vi "Special Replace of SubVI Node.vi"(6 "GObj Label":string, 8 "error in (no error)":errorcluster, 9 "Case Insensitive Match? (F)":bool, 10 "Class Path":path, 11 "vi reference in":refnum<vi>) -> (0 "error out":errorcluster, 2 "Replace":refnum<vi>, 3 "vi reference out":refnum<vi>)   [LabVIEW 2020, in "Message Maker.lvlib"]
uses:
  Message Maker.lvlib
  <vilib>/Utility/traverseref.llb/TRef TravTarget.ctl
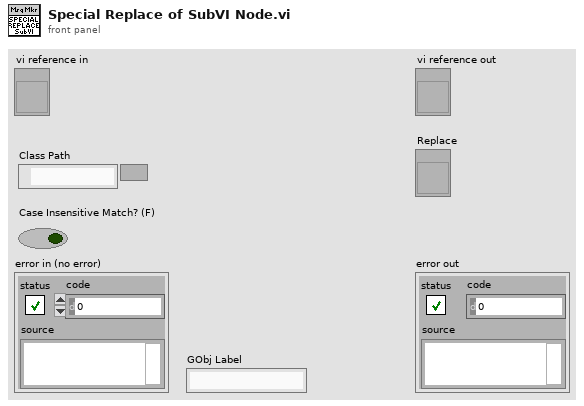
[diagram p1: front panel]
types:
  T1 = typedef "TRef TravTarget.ctl" = enum16{"FP", "BD", "Other"}
  T2 = typedef "LVPositionTypeDef.ctl" = cluster{"Left":i32, "Top":i32}
  T3 = typedef "LVBoundsTypeDef.ctl" = cluster{"Width":u32, "Height":u32}
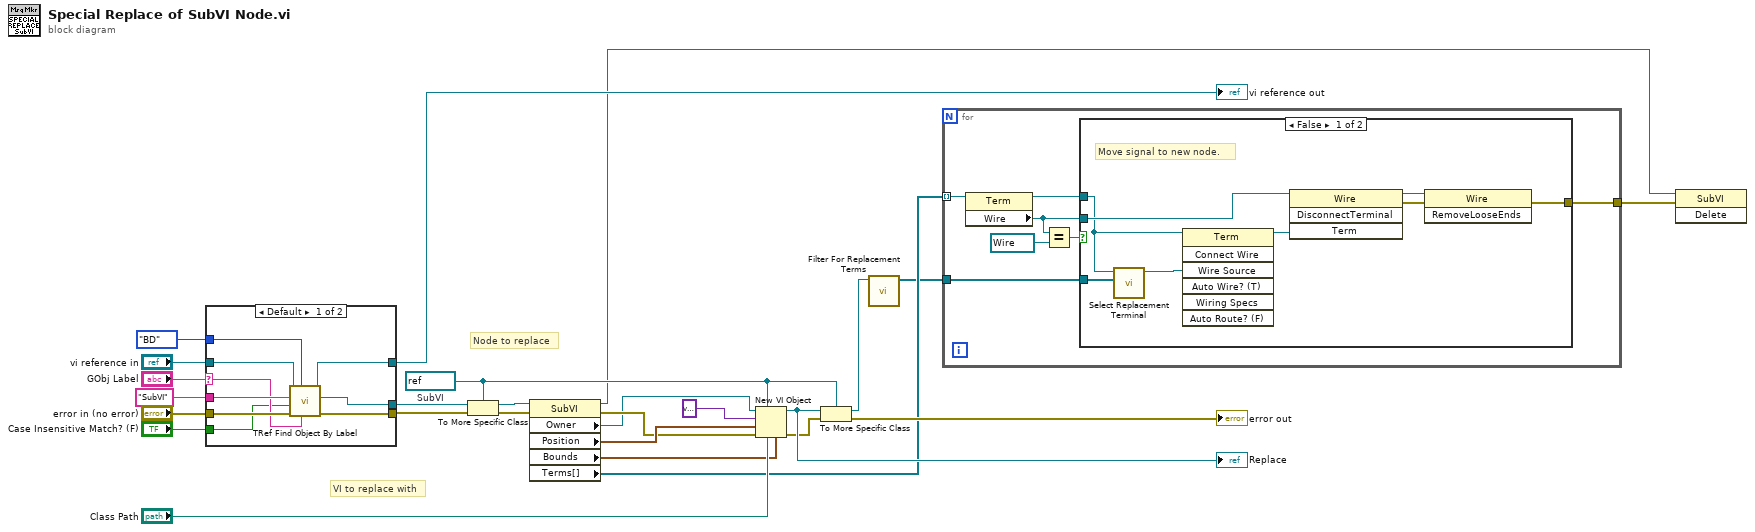
[diagram p0: block diagram]
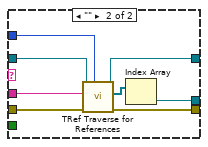
[diagram p2: hidden frame]
diagram:
  w7 = refnum<vi> refnum  # SubVI
  # "VI to replace with"
  # "Node to replace"
  n1 = case shown="Default" "GObj Label" {
    selector: "GObj Label" -> [w29 _]
    tunnel: [w34 w43] -> w17
    tunnel: [w28 w42] -> w19
    tunnel: "SubVI" ("GObj Class Name") -> [w30 w40]
    tunnel: TRef_TravTarget."BD" ("Traverse Target") -> [w33 w39]
    tunnel: [w31 w38] -> w24
    tunnel: "vi reference in" -> [w32 w37]
    tunnel: "error in (no error)" -> [w35 w36]
    tunnel: "Case Insensitive Match? (F)" -> [w27 _]
    frame Default {
      n2 = call <vilib>:"TRef Find Object By Label.vi"("Label"=w29, "Traverse Target"=w33, "error in (no error)"=w35, "Case Insensitive Match? (F)"=w27, "Class Name"=w30, "VI Ref"=w32) -> ("error out"=w34:errorcluster, "Found Obj Ref"=w28:refnum<vi>, "dup VI Ref"=w31:refnum<vi>)  [unwired: 2 in, 1 out]
    }
    frame "" {
      n3 = call <vilib>:"TRef Traverse for References.vi"("Traverse Target"=w39, "error in (no error)"=w36, "Class Name"=w40, "VI Refnum"=w37) -> ("error out"=w43:errorcluster, "References"=w41:refnum<vi>[], "dup VI Refnum"=w38:refnum<vi>)  [unwired: 4 in, 1 out]
      n4 = Index Array(array=w41) -> (element=w42:refnum<vi>)  [unwired: 1 in]
    }
  }
  "vi reference out" <- w24
  n5 = To More Specific Class(target class=w7, reference=w19, error in=w17) -> (specific class reference=w18:refnum<vi>, error out=w16:errorcluster)
  n6 = property class="SubVI"(reference=w18, error in=w16) -> (reference out=w2:refnum<vi>, error out=w15:errorcluster, "Owner"=w13:refnum<vi>, "Position"=w20:T2, "Bounds"=w11:T3, "Terms[]"=w6:refnum<vi>[])
  n7 = New VI Object(vi object class=w7, owner refnum=w13, style=variant, position/next to=w20, 4:w11, 6:"Class Path", 8:w15) -> (object refnum=w10:refnum<vi>, 0:w9:errorcluster)  [unwired: 1 in]
  "Replace" <- w10
  n8 = To More Specific Class(target class=w7, reference=w10, error in=w9) -> (specific class reference=w5:refnum<vi>, error out=→"error out":errorcluster)
  n9 = call "Filter For Replacement Terms.vi"("SubVI in"=w5) -> ("Terms[]"=w4:refnum<vi>[])  [unwired: 10 in]
  n10 = for {
    tunnel: w6 -> [w50] mode=indexing
    tunnel: w4 -> [w46]
    tunnel: [w44] -> w3
    n11 = property class="Term"(reference=w50) -> (reference out=w47:refnum<vi>, "Wire"=w45:refnum<vi>)  [unwired: 1 in, 1 out]
    n12 = Equal?(x=w45, y=refnum<vi> refnum ("Connected Wire")) -> (x = y?=w48:bool)
    n13 = case shown="False" w48 {
      tunnel: w47 -> [w51 _]
      tunnel: w46 -> [w58 _]
      tunnel: w45 -> [w57 _]
      tunnel: [w52 _] -> w44
      frame False {
        # "Move signal to new node."
        n14 = call "Select Replacement Terminal.vi"("Terms[]"=w58, "Terminal in"=w51) -> ("Terminal out"=w56:refnum<vi>)  [unwired: 9 in]
        n15 = invoke class="Term" method="Connect Wire"(reference=w51, "Wire Source"=w56) -> (reference out=w55:refnum<vi>)  [unwired: 5 in, 6 out]
        n16 = invoke class="Wire" method="DisconnectTerminal"(reference=w57, "Term"=w55) -> (reference out=w54:refnum<vi>, error out=w53:errorcluster)  [unwired: 2 in, 2 out]
        n17 = invoke class="Wire" method="RemoveLooseEnds"(reference=w54, error in=w53) -> (error out=w52:errorcluster)  [unwired: 1 in, 2 out]
      }
      frame True {
        # "Do nothing."
      }
    }
  }
  n18 = invoke class="SubVI" method="Delete"(reference=w2, error in=w3) -> ()  [unwired: 1 in, 3 out]
